vi "assenceur.vi"() -> ()   [LabVIEW 2017]
uses:
  Control 1.ctl
  <vilib>/Utility/miscctls.llb/LVPositionTypeDef.ctl
  <vilib>/Utility/miscctls.llb/LVBoundsTypeDef.ctl
panel:
  in  "Porte Ouverte":enum32{"Page 1"}(tab)
  in  "Porte Fermée":enum32{"Page 1"}(tab)
  in  "présence etage 2":bool
  in  "présence etage 1":bool
  in  "présence etage0":bool
  in  "Etage 2":bool
  in  "Etage 1":bool
  in  "Etage 0":bool
  in  "stop":bool
  in  "fermer la porte":bool
  out "App étage 0":bool
  out "App etage 1":bool
  out "App etage 2":bool
  in  "Ascenseur":dbl(slide) scale=0.0..10.0
  # "Paneau de control dans la cabine"
  # "Fermer la porte puis choisir une étage"
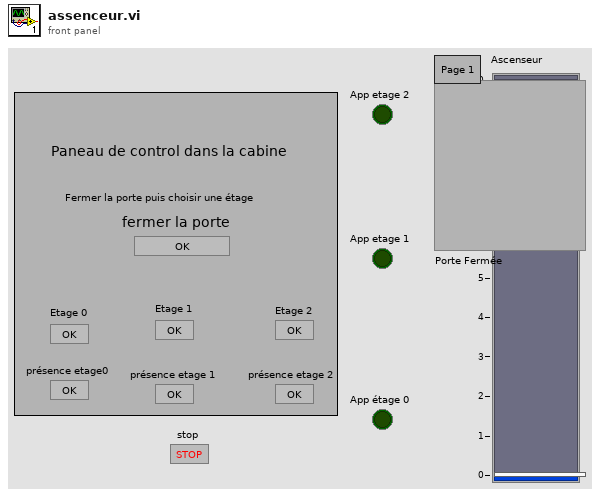
[diagram p1: front panel]
types:
  T1 = typedef "Control 1.ctl" = enum16{"init", "app ass", "presence etage0", "pressence etage1", "pressence etage2", "etage 0", "etage 1", "etage 2"}
  T2 = typedef "LVPositionTypeDef.ctl" = cluster{"Left":i32, "Top":i32}
  T3 = typedef "LVBoundsTypeDef.ctl" = cluster{"Width":u32, "Height":u32}
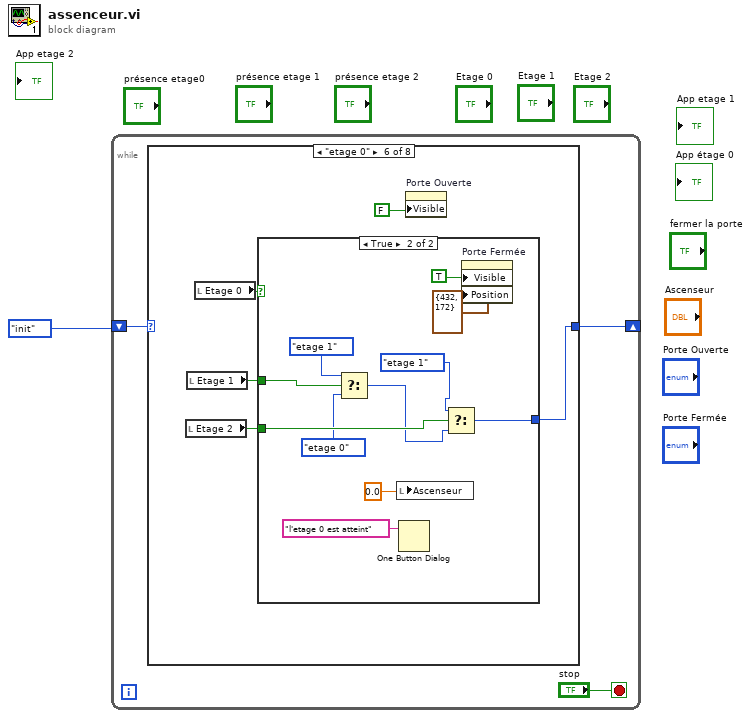
[diagram p0: block diagram]
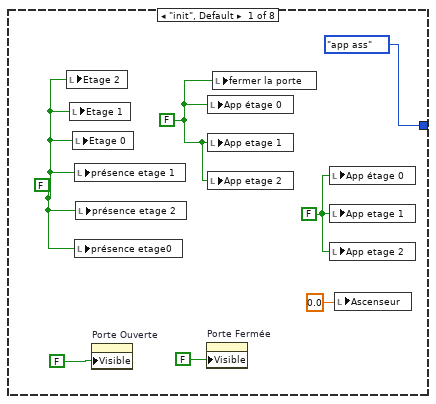
[diagram p2: hidden frame]
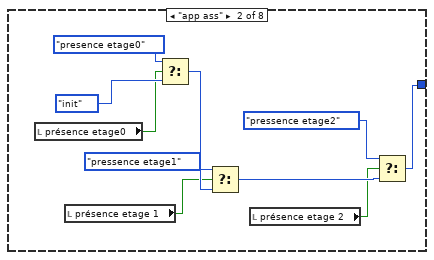
[diagram p3: hidden frame]
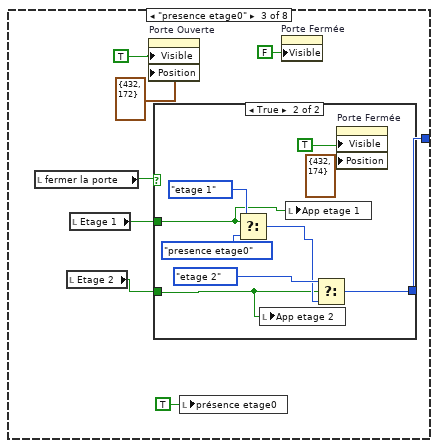
[diagram p4: hidden frame]
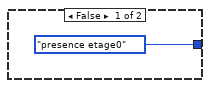
[diagram p5: hidden frame]
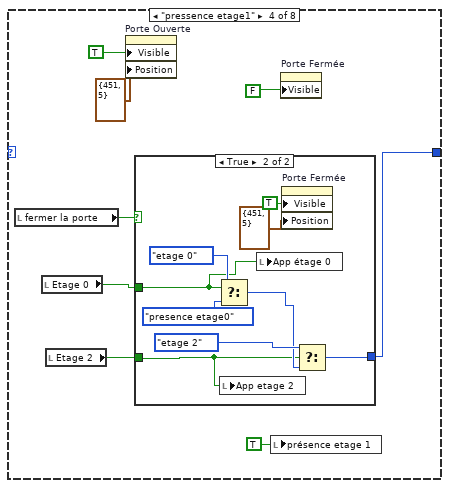
[diagram p6: hidden frame]
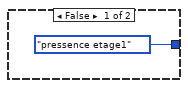
[diagram p7: hidden frame]
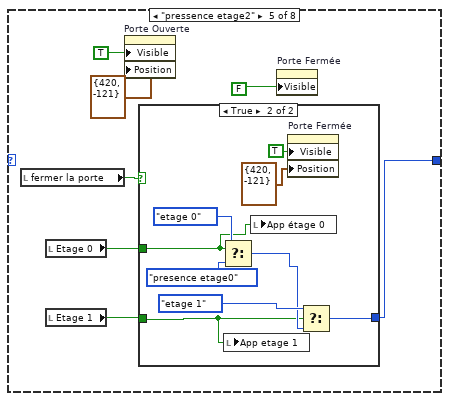
[diagram p8: hidden frame]
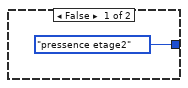
[diagram p9: hidden frame]
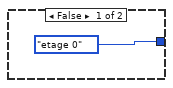
[diagram p10: hidden frame]
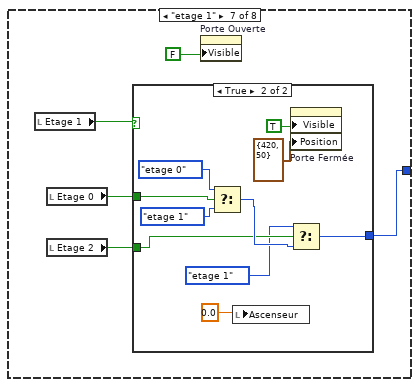
[diagram p11: hidden frame]
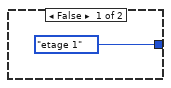
[diagram p12: hidden frame]
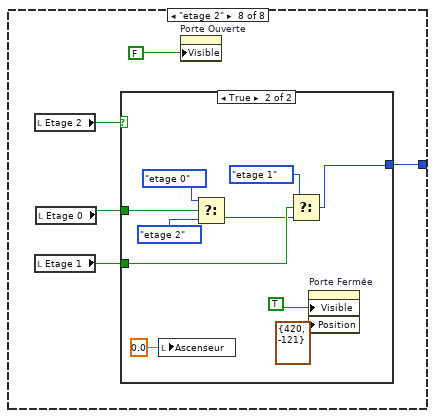
[diagram p13: hidden frame]
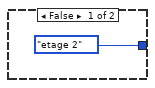
[diagram p14: hidden frame]
diagram:
  n1 = while {
    shift-right: [w2] -> _
    shift-left: Control_1."init" -> [w4]
    stop <- "stop" stop-if-true
    n2 = case shown="\"etage 0\"" w4 {
      tunnel: [Control_1."app ass" w12 w26 w44 w64 w76 w93 w109] -> w2
      frame "init", Default {
        w8 = FALSE
        w9 = FALSE
        w10 = FALSE ("etage 1")
        n3 = local write "Etage 2"(w9) -> ()
        n4 = local write "Etage 1"(w9) -> ()
        n5 = local write "Etage 0"(w9) -> ()
        n6 = local write "présence etage 1"(w9) -> ()
        n7 = local write "présence etage0"(w9) -> ()
        n8 = local write "présence etage 2"(w9) -> ()
        n9 = property on="Porte Ouverte" class="TabCtl (strict)"("Visible"=FALSE) -> ()  [unwired: 2 in, 2 out]
        n10 = property on="Porte Fermée" class="TabCtl (strict)"("Visible"=FALSE) -> ()  [unwired: 2 in, 2 out]
        n11 = local write "App étage 0"(w8) -> ()
        n12 = local write "App etage 1"(w8) -> ()
        n13 = local write "App etage 2"(w8) -> ()
        n14 = local write "fermer la porte"(w8) -> ()
        n15 = local write "App étage 0"(w10) -> ()
        n16 = local write "App etage 1"(w10) -> ()
        n17 = local write "App etage 2"(w10) -> ()
        n18 = local write "Ascenseur"(0.0 ("Slide")) -> ()
      }
      frame "app ass" {
        n19 = local read "présence etage0"() -> (w15:bool)
        n20 = local read "présence etage 1"() -> (w14:bool)
        n21 = Select(t=Control_1."presence etage0", s=w15, f=Control_1."init") -> (s? t:f=w16:T1)
        n22 = Select(t=Control_1."pressence etage1", s=w14, f=w16) -> (s? t:f=w20:T1)
        n23 = local read "présence etage 2"() -> (w13:bool)
        n24 = Select(t=Control_1."pressence etage2", s=w13, f=w20) -> (s? t:f=w12:T1)
      }
      frame "presence etage0" {
        n25 = local read "fermer la porte"() -> (w29:bool)
        n26 = local read "Etage 2"() -> (w27:bool)
        n27 = local read "Etage 1"() -> (w28:bool)
        n28 = property on="Porte Ouverte" class="TabCtl (strict)"("Visible"=TRUE, "Position"=T2 {"Left"=432, "Top"=172}) -> ()  [unwired: 2 in, 2 out]
        n29 = case shown="True" w29 {
          tunnel: w28 -> [_ w34]
          tunnel: w27 -> [_ w33]
          tunnel: [Control_1."presence etage0" w35] -> w26
          frame False {
          }
          frame True {
            n30 = Select(t=Control_1."etage 1", s=w34, f=Control_1."presence etage0") -> (s? t:f=w36:T1)
            n31 = local write "App etage 2"(w33) -> ()
            n32 = local write "App etage 1"(w34) -> ()
            n33 = Select(t=Control_1."etage 2", s=w33, f=w36) -> (s? t:f=w35:T1)
            n34 = property on="Porte Fermée" class="TabCtl (strict)"("Visible"=TRUE, "Position"=T3 {"Width"=432, "Height"=174} ("Bounds")) -> ()  [unwired: 2 in, 2 out]
          }
        }
        n35 = local write "présence etage0"(TRUE ("présence etage0")) -> ()
        n36 = property on="Porte Fermée" class="TabCtl (strict)"("Visible"=FALSE) -> ()  [unwired: 2 in, 2 out]
      }
      frame "pressence etage1" {
        n37 = local read "fermer la porte"() -> (w47:bool)
        n38 = local read "Etage 0"() -> (w46:bool)
        n39 = local read "Etage 2"() -> (w45:bool)
        n40 = property on="Porte Ouverte" class="TabCtl (strict)"("Visible"=TRUE, "Position"=T2 {"Left"=451, "Top"=5}) -> ()  [unwired: 2 in, 2 out]
        n41 = case shown="True" w47 {
          tunnel: w46 -> [_ w51]
          tunnel: w45 -> [_ w52]
          tunnel: [Control_1."pressence etage1" w53] -> w44
          frame False {
          }
          frame True {
            n42 = Select(t=Control_1."etage 0", s=w51, f=Control_1."presence etage0") -> (s? t:f=w54:T1)
            n43 = local write "App etage 2"(w52) -> ()
            n44 = local write "App étage 0"(w51) -> ()
            n45 = property on="Porte Fermée" class="TabCtl (strict)"("Visible"=TRUE, "Position"=T2 {"Left"=451, "Top"=5}) -> ()  [unwired: 2 in, 2 out]
            n46 = Select(t=Control_1."etage 2", s=w52, f=w54) -> (s? t:f=w53:T1)
          }
        }
        n47 = local write "présence etage 1"(TRUE ("présence etage 1")) -> ()
        n48 = property on="Porte Fermée" class="TabCtl (strict)"("Visible"=FALSE) -> ()  [unwired: 2 in, 2 out]
      }
      frame "pressence etage2" {
        n49 = local read "fermer la porte"() -> (w63:bool)
        n50 = local read "Etage 0"() -> (w62:bool)
        n51 = local read "Etage 1"() -> (w61:bool)
        n52 = property on="Porte Ouverte" class="TabCtl (strict)"("Visible"=TRUE, "Position"=T2 {"Left"=420, "Top"=-121}) -> ()  [unwired: 2 in, 2 out]
        n53 = case shown="True" w63 {
          tunnel: w62 -> [_ w69]
          tunnel: w61 -> [_ w68]
          tunnel: [Control_1."pressence etage2" w70] -> w64
          frame False {
          }
          frame True {
            n54 = Select(t=Control_1."etage 0", s=w69, f=Control_1."presence etage0") -> (s? t:f=w71:T1)
            n55 = local write "App etage 1"(w68) -> ()
            n56 = local write "App étage 0"(w69) -> ()
            n57 = property on="Porte Fermée" class="TabCtl (strict)"("Visible"=TRUE, "Position"=T2 {"Left"=420, "Top"=-121}) -> ()  [unwired: 2 in, 2 out]
            n58 = Select(t=Control_1."etage 1", s=w68, f=w71) -> (s? t:f=w70:T1)
          }
        }
        n59 = property on="Porte Fermée" class="TabCtl (strict)"("Visible"=FALSE) -> ()  [unwired: 2 in, 2 out]
      }
      frame "etage 0" {
        n60 = local read "Etage 2"() -> (w77:bool)
        n61 = local read "Etage 1"() -> (w78:bool)
        n62 = local read "Etage 0"() -> (w79:bool)
        n63 = case shown="True" w79 {
          tunnel: w78 -> [_ w90]
          tunnel: w77 -> [_ w89]
          tunnel: [Control_1."etage 0" w84] -> w76
          frame False {
          }
          frame True {
            n64 = Select(t=Control_1."etage 1", s=w90, f=Control_1."etage 0") -> (s? t:f=w88:T1)
            n65 = local write "Ascenseur"(0.0 ("Slide")) -> ()
            n66 = One Button Dialog(message="l'etage 0 est atteint") -> ()  [unwired: 1 in, 1 out]
            n67 = Select(t=Control_1."etage 1", s=w89, f=w88) -> (s? t:f=w84:T1)
            n68 = property on="Porte Fermée" class="TabCtl (strict)"("Visible"=TRUE, "Position"=T2 {"Left"=432, "Top"=172}) -> ()  [unwired: 2 in, 2 out]
          }
        }
        n69 = property on="Porte Ouverte" class="TabCtl (strict)"("Visible"=FALSE) -> ()  [unwired: 2 in, 2 out]
      }
      frame "etage 1" {
        n70 = local read "Etage 1"() -> (w96:bool)
        n71 = local read "Etage 0"() -> (w95:bool)
        n72 = local read "Etage 2"() -> (w94:bool)
        n73 = case shown="True" w96 {
          tunnel: w95 -> [_ w105]
          tunnel: w94 -> [_ w106]
          tunnel: [Control_1."etage 1" w101] -> w93
          frame False {
          }
          frame True {
            n74 = Select(t=Control_1."etage 0", s=w105, f=Control_1."etage 1") -> (s? t:f=w107:T1)
            n75 = local write "Ascenseur"(0.0 ("Slide")) -> ()
            n76 = property on="Porte Fermée" class="TabCtl (strict)"("Visible"=TRUE, "Position"=T2 {"Left"=420, "Top"=50}) -> ()  [unwired: 2 in, 2 out]
            n77 = Select(t=Control_1."etage 1", s=w106, f=w107) -> (s? t:f=w101:T1)
          }
        }
        n78 = property on="Porte Ouverte" class="TabCtl (strict)"("Visible"=FALSE) -> ()  [unwired: 2 in, 2 out]
      }
      frame "etage 2" {
        n79 = local read "Etage 2"() -> (w112:bool)
        n80 = local read "Etage 1"() -> (w110:bool)
        n81 = local read "Etage 0"() -> (w111:bool)
        n82 = case shown="True" w112 {
          tunnel: w111 -> [_ w123]
          tunnel: w110 -> [_ w122]
          tunnel: [Control_1."etage 2" w117] -> w109
          frame False {
          }
          frame True {
            n83 = local write "Ascenseur"(0.0 ("Slide")) -> ()
            n84 = Select(t=Control_1."etage 0", s=w123, f=Control_1."etage 2") -> (s? t:f=w118:T1)
            n85 = Select(t=Control_1."etage 1", s=w122, f=w118) -> (s? t:f=w117:T1)
            n86 = property on="Porte Fermée" class="TabCtl (strict)"("Visible"=TRUE, "Position"=T2 {"Left"=420, "Top"=-121}) -> ()  [unwired: 2 in, 2 out]
          }
        }
        n87 = property on="Porte Ouverte" class="TabCtl (strict)"("Visible"=FALSE) -> ()  [unwired: 2 in, 2 out]
      }
    }
  }
